vi "SetTo0.vi"(10 "Longueur d'onde":dbl) -> (2 "Température 0":dbl)   [LabVIEW 2018]
uses:
  <vilib>/DAQmx/write.llb/DAQmx Write (Digital 1D Bool NChan 1Samp 1Line).vi
  <vilib>/DAQmx/read.llb/DAQmx Read (Analog 1D Wfm NChan NSamp).vi
  <vilib>/Analysis/baseanly.llb/Mean (DBL).vi
  <vilib>/DAQmx/create/channels.llb/DAQmx Create Channel (DO-Digital Output).vi
  <vilib>/DAQmx/miscellaneous.llb/DAQmx Fill In Error Info.vi
  <vilib>/DAQmx/create/channels.llb/DAQmx Create Channel (AI-Voltage-Basic).vi
  <vilib>/DAQmx/configure/timing.llb/DAQmx Timing (Sample Clock).vi
  <vilib>/Analysis/NI_AALBase.lvlib
  <resource>/objmgr/daqmx.rc
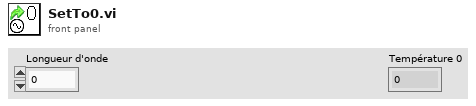
[diagram p1: front panel]
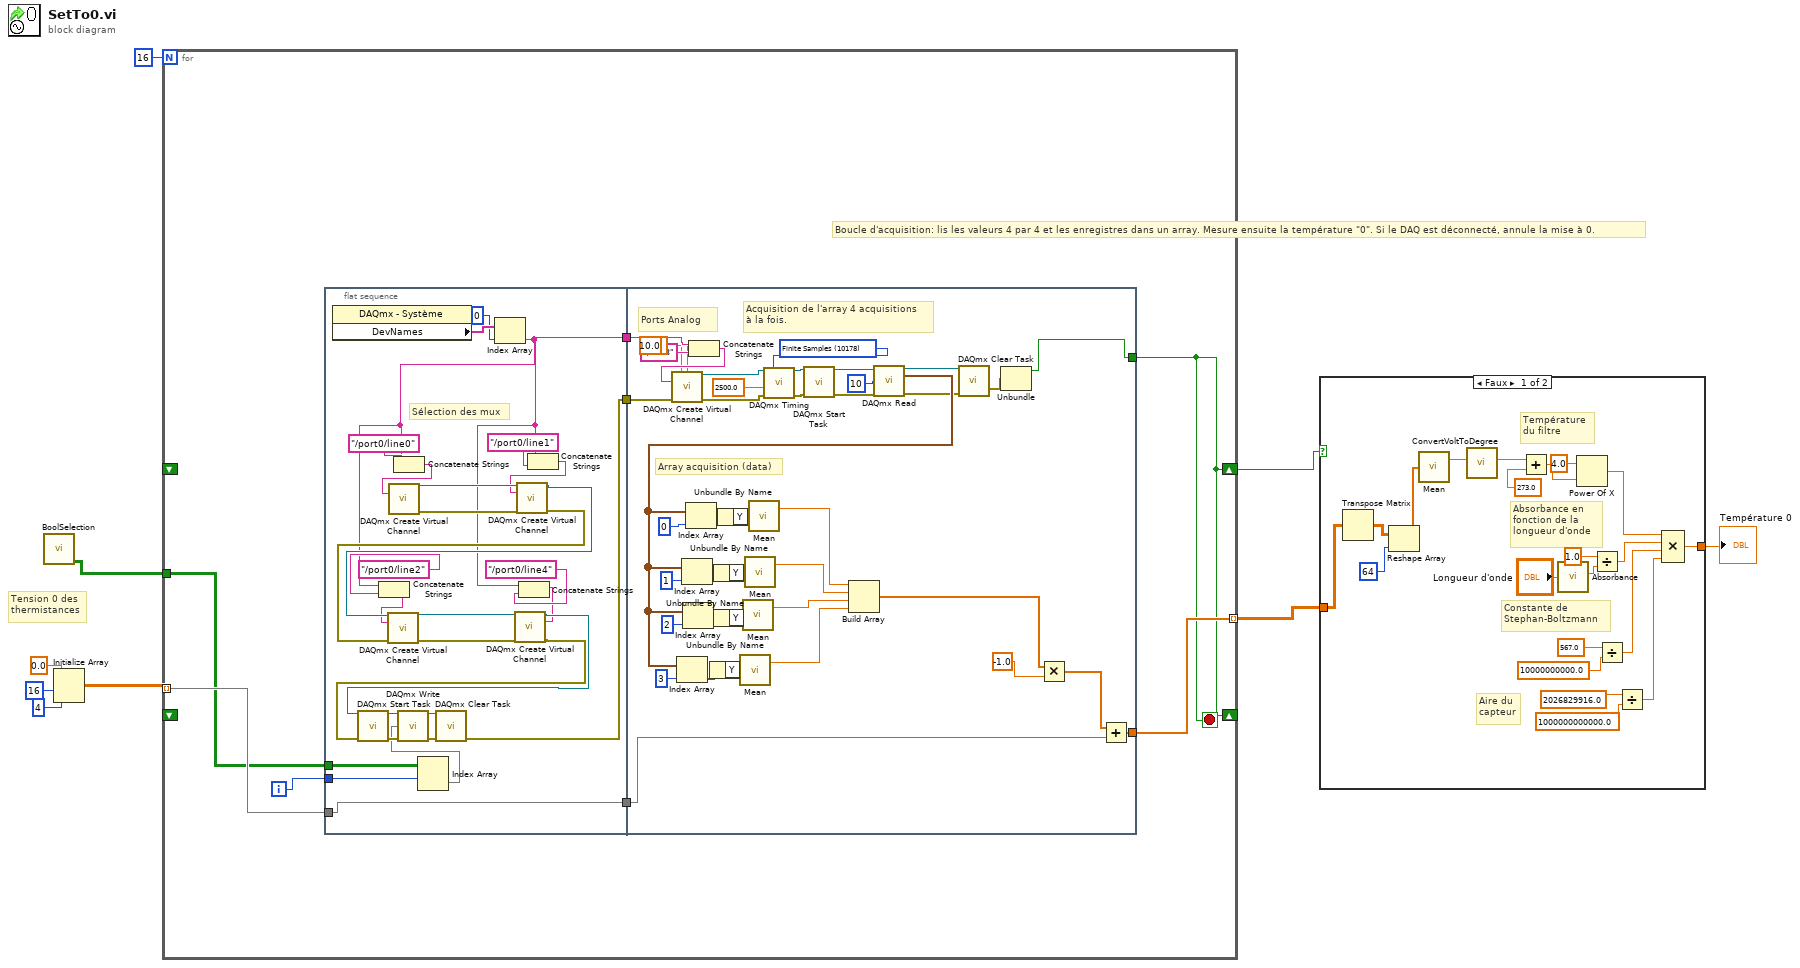
[diagram p0: block diagram]
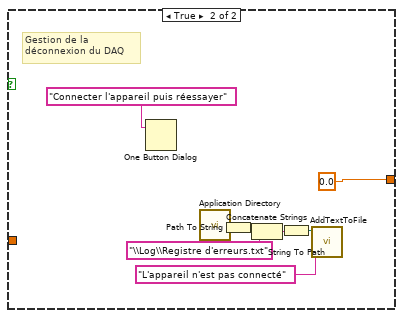
[diagram p2: hidden frame]
diagram:
  # "Tension 0 des \nthermistances"
  # "Boucle d'acquisition: lis les valeurs 4 par 4 et les enregistres dans un array. Mesure ensuite la température \"0\". Si le DAQ est déconnecté, annule la mise à 0."
  n1 = call "BoolSelection.vi"() -> ("BoolSelection"=w1:bool[][])  [unwired: 11 in]
  n2 = Initialize Array(0.0 ("element"), 16 ("dimension size"), 4 ("dimension size")) -> (w2:dbl[][])
  n3 = for {
    N: 16 -> [_]
    tunnel: w1 -> [w12]
    tunnel: w2 -> [w17] mode=indexing
    tunnel: [w11] -> w7 mode=indexing
    shift-right: [w10] -> _
    shift-left: _ -> [_]
    shift-right: [w10] -> w8
    shift-left: _ -> [_]
    i -> [w13]
    stop <- w10 stop-if-true
    n4 = flat-sequence {
      tunnel: w13 -> [w31]
      tunnel: [w42] -> w16
      tunnel: w12 -> [w30]
      tunnel: [w18] -> w15
      tunnel: [w19] -> w14
      tunnel: w17 -> [w18]
      tunnel: w16 -> [w78]
      tunnel: w15 -> [w59]
      tunnel: [w60] -> w11
      tunnel: w14 -> [w56]
      tunnel: [w51] -> w10
      frame #0 {
        # "Sélection des mux"
        n5 = property class="DAQmx - Système"() -> ("DevNames"=w29:tag[])  [unwired: 2 in, 2 out]
        n6 = Index Array(array=w30, index (row)=w31) -> (element=w43:bool[])  [unwired: 1 in]
        n7 = Index Array(array=w29, index=0) -> (element=w19:tag)
        n8 = Concatenate Strings(w19, "/port0/line2" ("string")) -> (w22:string)
        n9 = Concatenate Strings(w19, "/port0/line0" ("string")) -> (w27:string)
        n10 = call-poly <vilib>:"DAQmx Create Virtual Channel.vi"("lines"=w27) -> ("task out"=w38:refnum<k21>, "error out"=w39:errorcluster)  [unwired: 13 in]
        n11 = Concatenate Strings(w19, "/port0/line4" ("string")) -> (w20:string)
        n12 = Concatenate Strings(w19, "/port0/line1" ("string")) -> (w24:string)
        n13 = call-poly <vilib>:"DAQmx Create Virtual Channel.vi"("task in"=w38, "lines"=w24, "error in"=w39) -> ("task out"=w37:refnum<k21>, "error out"=w36:errorcluster)  [unwired: 11 in]
        n14 = call-poly <vilib>:"DAQmx Create Virtual Channel.vi"("task in"=w37, "lines"=w22, "error in"=w36) -> ("task out"=w34:refnum<k21>, "error out"=w35:errorcluster)  [unwired: 11 in]
        n15 = call-poly <vilib>:"DAQmx Create Virtual Channel.vi"("task in"=w34, "lines"=w20, "error in"=w35) -> ("task out"=w33:refnum<k21>, "error out"=w32:errorcluster)  [unwired: 11 in]
        n16 = call <vilib>:"DAQmx Start Task.vi"("task/channels in"=w33, "error in"=w32) -> ("task out"=w44:refnum<k21>, "error out"=w45:errorcluster)  [unwired: 12 in]
        n17 = call-poly <vilib>:"DAQmx Write.vi"("task/channels in"=w44, "data"=w43, "error in"=w45) -> ("task out"=w41:refnum<k21>, "error out"=w40:errorcluster)  [unwired: 10 in, 1 out]
        n18 = call <vilib>:"DAQmx Clear Task.vi"("task in"=w41, "error in"=w40) -> ("error out"=w42:errorcluster)  [unwired: 13 in]
      }
      frame #1 {
        w80 = 10178 items=["Finite Samples"=10178, "Continuous Samples"=10123, "Hardware Timed Single Point"=12522] ("sample mode")
        # "Ports Analog"
        # "Array acquisition (data)"
        # "Acquisition de l'array 4 acquisitions\nà la fois."
        n19 = Concatenate Strings(w56, "/ai0:3" ("string")) -> (w57:string)
        n20 = call-poly <vilib>:"DAQmx Create Virtual Channel.vi"("maximum value"=10.0, "minimum value"=-10.0, "physical channels"=w57, "error in"=w78) -> ("task out"=w85:refnum<k21>, "error out"=w84:errorcluster)  [unwired: 10 in]
        n21 = call-poly <vilib>:"DAQmx Timing.vi"("task/channels in"=w85, "sample mode"=w80, "rate"=2500.0, "error in"=w84) -> ("task out"=w81:refnum<k21>, "error out"=w82:errorcluster)  [unwired: 10 in]
        n22 = call <vilib>:"DAQmx Start Task.vi"("task/channels in"=w81, "error in"=w82) -> ("task out"=w83:refnum<k21>, "error out"=w86:errorcluster)  [unwired: 12 in]
        n23 = call-poly <vilib>:"DAQmx Read.vi"("task/channels in"=w83, "number of samples per channel"=10, "error in"=w86) -> ("task out"=w62:refnum<k21>, "data"=w71:waveform(dbl)[], "error out"=w61:errorcluster)  [unwired: 10 in]
        n24 = Index Array(array=w71, index=3) -> (element=w67:waveform(dbl))
        n25 = Index Array(array=w71, index=1) -> (element=w69:waveform(dbl))
        n26 = Index Array(array=w71, index=2) -> (element=w68:waveform(dbl))
        n27 = Index Array(array=w71, index=0) -> (element=w70:waveform(dbl))
        n28 = Unbundle By Name(w67) -> ("Y"=w63:dbl[])
        n29 = Unbundle By Name(w69) -> ("Y"=w65:dbl[])
        n30 = Unbundle By Name(w68) -> ("Y"=w64:dbl[])
        n31 = Unbundle By Name(w70) -> ("Y"=w66:dbl[])
        n32 = call-poly <vilib>:"Mean.vi"("X"=w63) -> ("mean"=w52:dbl)  [unwired: 1 out]
        n33 = call-poly <vilib>:"Mean.vi"("X"=w64) -> ("mean"=w53:dbl)  [unwired: 1 out]
        n34 = call-poly <vilib>:"Mean.vi"("X"=w65) -> ("mean"=w54:dbl)  [unwired: 1 out]
        n35 = call-poly <vilib>:"Mean.vi"("X"=w66) -> ("mean"=w55:dbl)  [unwired: 1 out]
        n36 = Build Array(w55, w54, w53, w52) -> (w46:dbl[])
        n37 = call <vilib>:"DAQmx Clear Task.vi"("task in"=w62, "error in"=w61) -> ("error out"=w76:errorcluster)  [unwired: 13 in]
        n38 = Unbundle(w76) -> ("status"=w51:bool)  [unwired: 2 out]
        n39 = Multiply(x=w46, y=-1.0) -> (x*y=w47:dbl[])
        n40 = Add(x=w47, y=w59) -> (x+y=w60:dbl[])
      }
    }
  }
  n41 = case shown="Faux" w8 {
    tunnel: w7 -> [w94 _]
    tunnel: [w90 0.0] -> w9
    frame False {
      # "Constante de \nStephan-Boltzmann"
      # "Absorbance en\nfonction de la \nlongueur d'onde"
      # "Température \ndu filtre"
      # "Aire du\ncapteur"
      n42 = Transpose Matrix(1:w94) -> (0:w95:dbl[][])
      n43 = Reshape Array(w95, 64 ("dimension size")) -> (w92:dbl[])
      n44 = call-poly <vilib>:"Mean.vi"("X"=w92) -> ("mean"=w91:dbl)  [unwired: 1 out]
      n45 = call "ConvertVoltToDegree.vi"("Tension"=w91) -> ("Température"=w99:dbl)  [unwired: 10 in]
      n46 = Add(x=w99, y=273.0) -> (x+y=w106:dbl)
      n47 = call "Absorbance.vi"("Longueur d'onde"="Longueur d'onde") -> ("absorbance"=w88:dbl)  [unwired: 10 in]
      n48 = Power Of X(1:w106, 2:4.0 ("y")) -> (0:w96:dbl)
      n49 = Divide(x=1.0, y=w88) -> (x/y=w89:dbl)
      n50 = Divide(x=567.0, y=10000000000.0) -> (x/y=w97:dbl)
      n51 = Divide(x=2026829916.0, y=1000000000000.0) -> (x/y=w98:dbl)
      n52 = Compound Arithmetic op=MULTIPLY(w96, w89, w97, w98) -> (w90:dbl)
    }
    frame True {
      # "Gestion de la \ndéconnexion du DAQ"
      n53 = One Button Dialog(message="Connecter l'appareil puis réessayer") -> ()  [unwired: 1 in, 1 out]
      n54 = call <vilib>:"Application Directory.vi"() -> ("Application Directory"=w111:path)
      n55 = Path To String(path=w111) -> (string=w112:string)
      n56 = Concatenate Strings(w112, "\\Log\\Registre d'erreurs.txt") -> (w113:string)
      n57 = String To Path(string=w113) -> (path=w109:path)
      n58 = call "AddTextToFile.vi"("Ajouter du texte"="L'appareil n'est pas connecté", "Fichier"=w109) -> ()  [unwired: 10 in]
    }
  }
  "Température 0" <- w9
